vi "PostTeamsToDatabase.vi"(8 "error in (no error)":errorcluster) -> (0 "error out":errorcluster)   [LabVIEW 2014, in "FIRST Events API.lvlib"]
uses:
  FIRST Events API.lvlib
  Backend/source/VI Source/FRCts20_Backend_API/FRCts20_Backend_API_Command_TeamRoot.ctl
  Backend/source/VI Source/FRCts20_Backend_API/FRCts20_Backend_API_TeamRoot.ctl
  Backend/source/VI Source/FRCts20_Backend_API/FRCts20_Backend_API_SW.ctl
  Backend/source/VI Source/FRCts20_Backend_API/FRCts20_Backend_API_TeamRoot.vi
  Backend/source/VI Source/FRCts20_Backend_API/FRCts20_Backend_API.lvlib
panel:
  out "Items Added to Database":i32
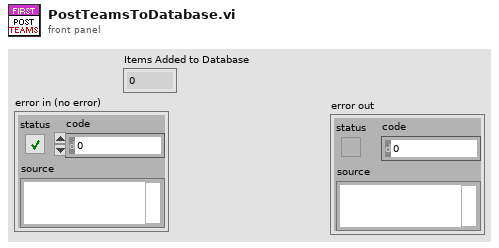
[diagram p1: front panel]
types:
  T1 = typedef "FRCts20_Backend_API.lvlib/FRCts20_Backend_API_TeamRoot.ctl" = cluster{"Teams":cluster{"Team Index":u32, "Team Number":u32, "Team ID":u32, "Team Name":string, "Short Team Name":string, "Nick Name":string, "Robot Name":string, "City":string, "State":string, "Country":string, "Rookie Year":u32, "SWType":T2, "CAN":bool, "Vision":bool, "Kinect":bool, "Tags":string, "Avatar":string, "Events":cluster{"EventIndex":u32, "EventName":string, "IsLive":bool}[]}[], "APIReturn":string}
  T2 = typedef "FRCts20_Backend_API.lvlib/FRCts20_Backend_API_SW.ctl" = string
  T3 = typedef "FRCts20_Backend_API.lvlib/FRCts20_Backend_API_Command_TeamRoot.ctl" = string
  T4 = cluster{"Team Index":u32, "Team Number":u32, "Team ID":u32, "Team Name":string, "Short Team Name":string, "Nick Name":string, "Robot Name":string, "City":string, "State":string, "Country":string, "Rookie Year":u32, "SWType":T2, "CAN":bool, "Vision":bool, "Kinect":bool, "Tags":string, "Avatar":string, "Events":cluster{"EventIndex":u32, "EventName":string, "IsLive":bool}[]}[]
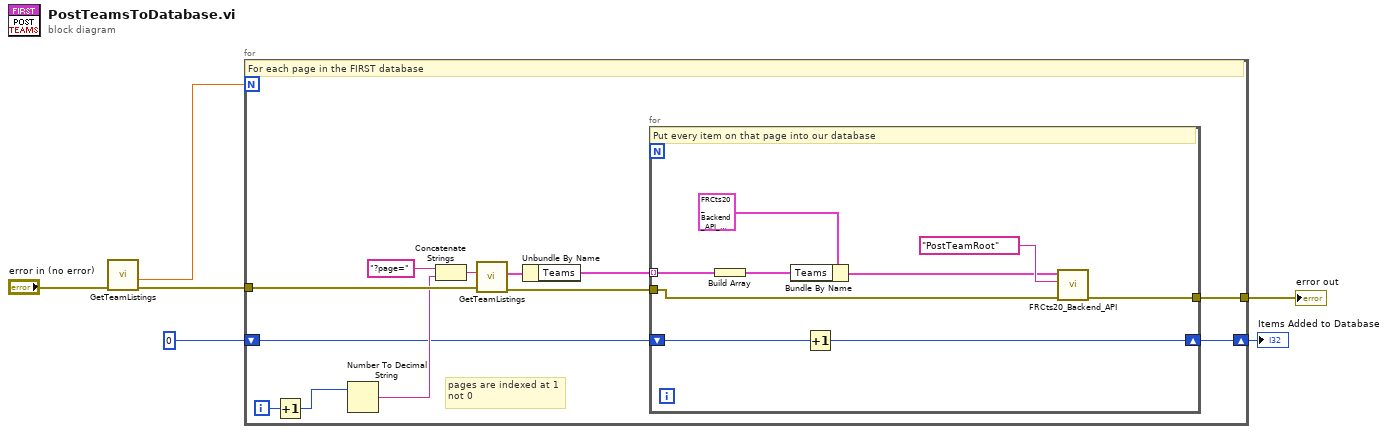
[diagram p0: block diagram]
diagram:
  n1 = call "GetTeamListings.vi"("error in (no error)"="error in (no error)") -> ("error out"=w6:errorcluster, "pageTotal"=w5:dbl)  [unwired: 8 in, 1 out]
  n2 = for {
    N: w5 -> [_]
    tunnel: w6 -> [w17]
    tunnel: [w9] -> w4
    shift-right: [w7] -> w2
    shift-left: 0 ("Numeric") -> [w8]
    i -> [w18]
    # "pages are indexed at 1\nnot 0"
    # "For each page in the FIRST database"
    n3 = Increment(x=w18) -> (x+1=w16:i32)
    n4 = Number To Decimal String(number=w16) -> (decimal integer string=w14:string)  [unwired: 1 in]
    n5 = Concatenate Strings("?page=" ("string"), w14) -> (w15:string)
    n6 = call "GetTeamListings.vi"("error in (no error)"=w17, "Append to URL"=w15) -> ("error out"=w12:errorcluster, "output cluster"=w11:T1)  [unwired: 7 in, 1 out]
    n7 = Unbundle By Name(w11) -> ("Teams"=w10:T4)
    n8 = for {
      tunnel: w12 -> [w22]
      tunnel: w10 -> [w24] mode=indexing
      tunnel: [w21] -> w9
      shift-right: [w19] -> w7
      shift-left: w8 -> [w20]
      # "Put every item on that page into our database"
      n9 = Build Array(w24) -> (w26:T4)
      n10 = Bundle By Name(cluster=T1 {"Teams"=[{"Team Index"=0, "Team Number"=0, "Team ID"=0, "Team Name"="", "Short Team Name"="", "Nick Name"="", "Robot Name"="", "City"="", "State"="", "Country"="", "Rookie Year"=0, "SWType"="unknown", "CAN"=FALSE, "Vision"=FALSE, "Kinect"=FALSE, "Tags"="", "Avatar"="", "Events"=[]}], "APIReturn"=""} ("output cluster"), "Teams"=w26) -> (w23:T1)
      n11 = Increment(x=w20) -> (x+1=w19:i32)
      n12 = call-poly "FRCts20_Backend_API.vi"("error in (no error)"=w22, "Command"=T3 "PostTeamRoot", "Team In"=w23) -> ("error out"=w21:errorcluster)  [unwired: 6 in, 2 out]
    }
  }
  "error out" <- w4
  "Items Added to Database" <- w2
